vi "HW XML Tx - Write.vi"(0 "String (in)":string, 7 "Parameter Array":T1[](array[typedef])) -> (4 "String (out)":string)   [LabVIEW 2017]
uses:
  Controls/Database_Array.ctl
  Controls/Encoding.ctl
  <userlib>/_OpenG.lib/array/array.llb/Remove Duplicates from 1D Array (I32)__ogtk.vi
  <userlib>/_OpenG.lib/array/array.llb/Filter 1D Array with Scalar (I32)__ogtk.vi
  <userlib>/_OpenG.lib/array/array.llb/Index 1D Array Elements (Variant)__ogtk.vi
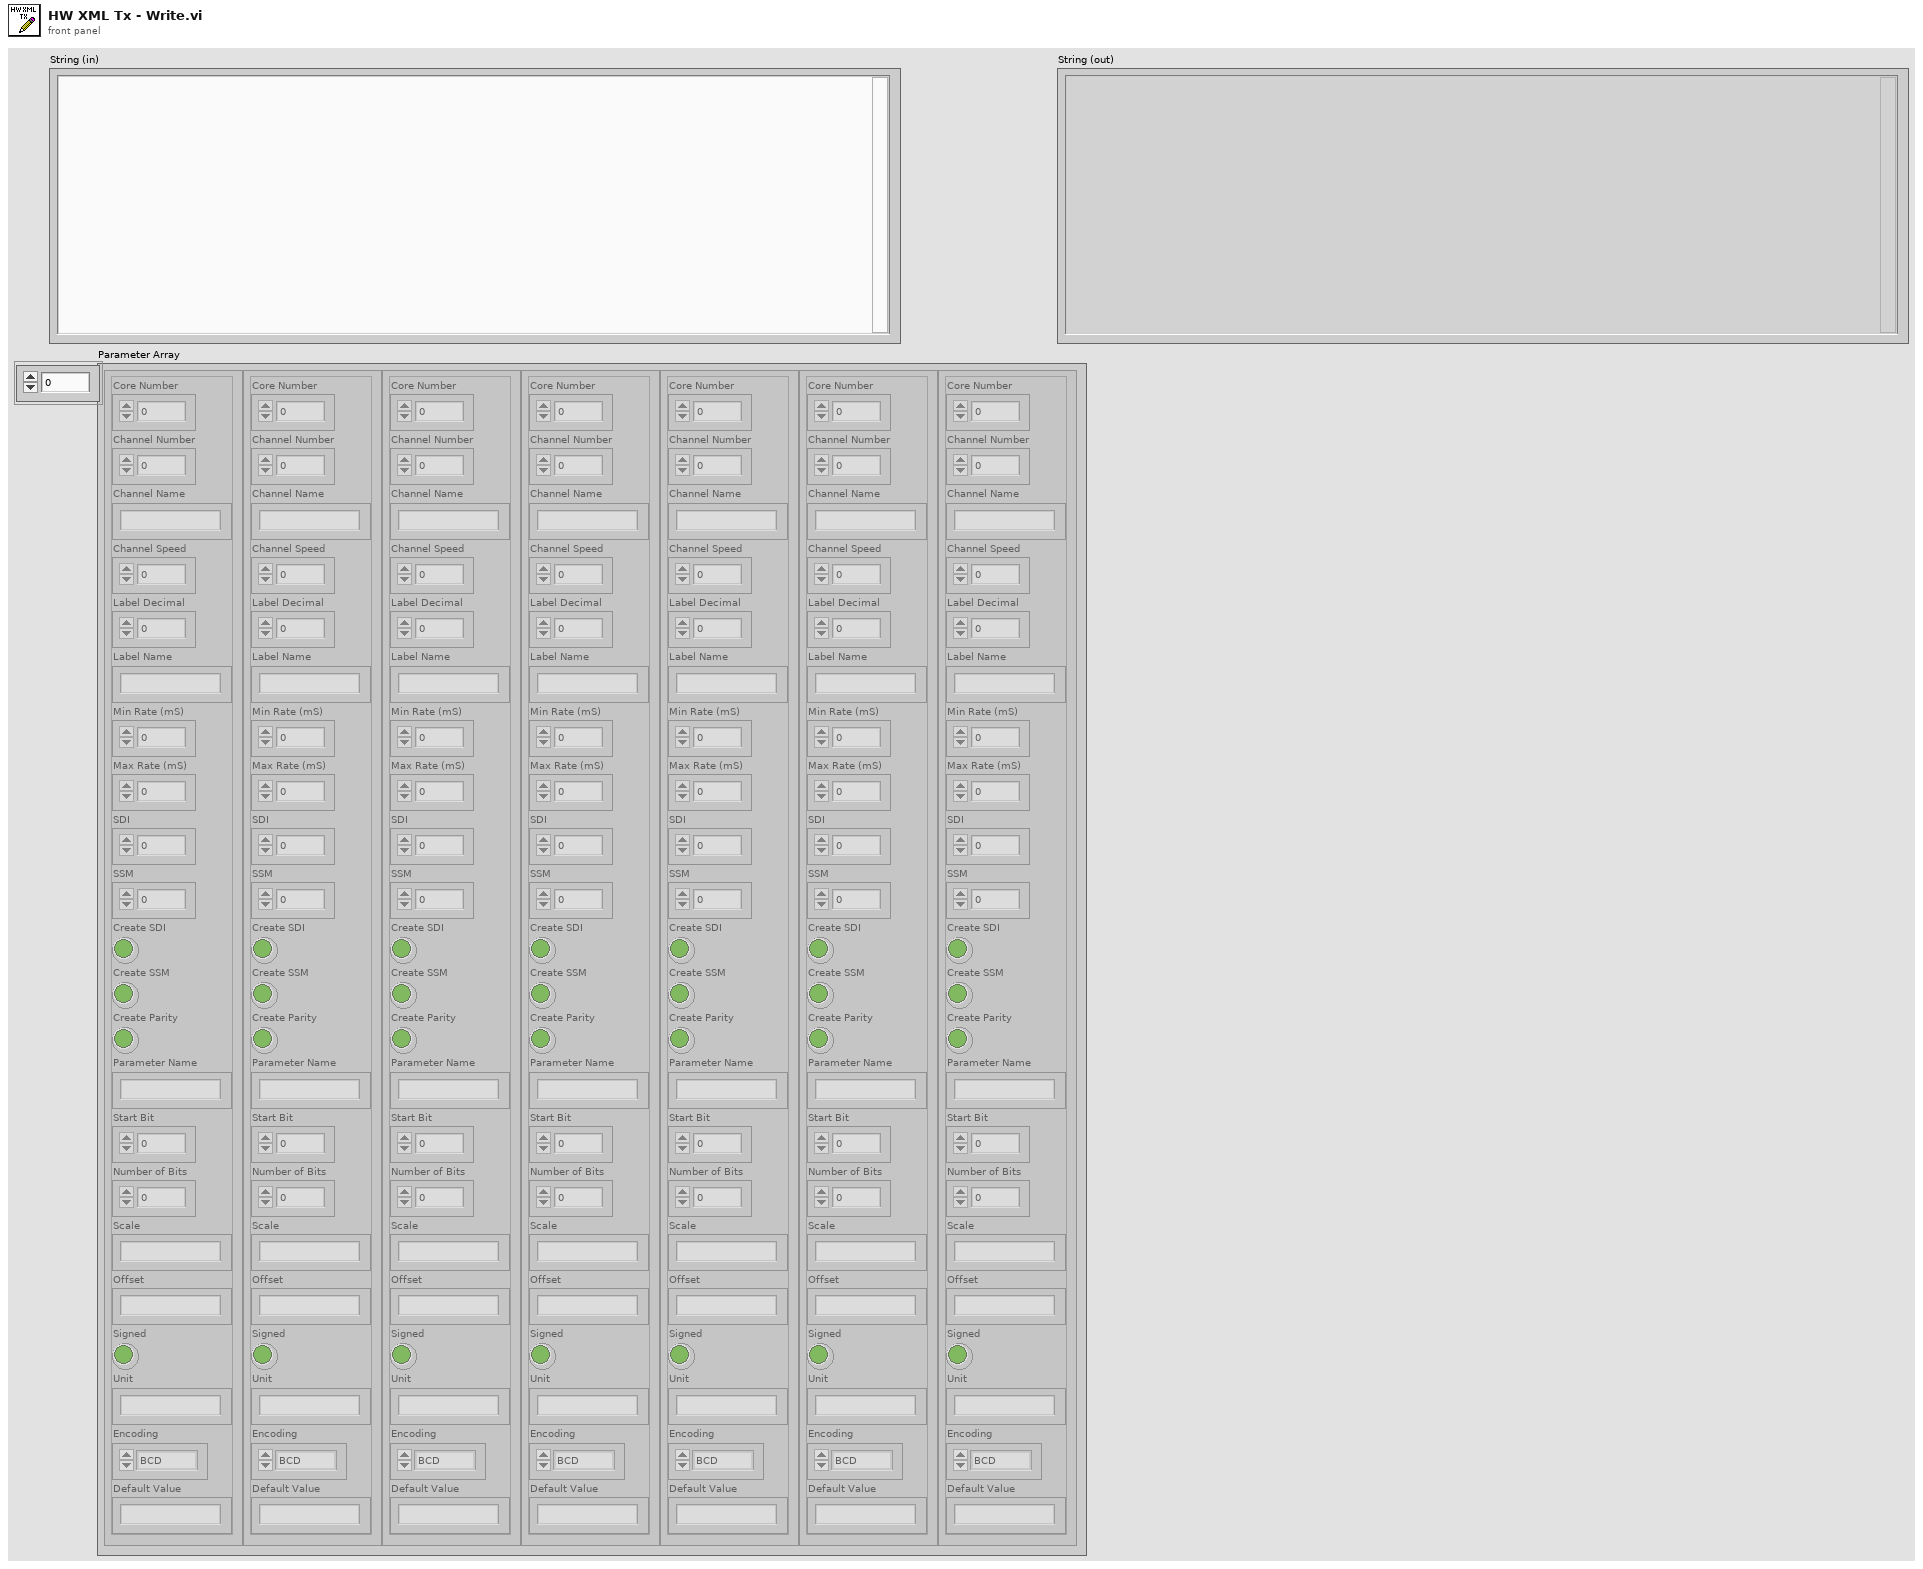
[diagram p1: front panel]
types:
  T1 = typedef "Database_Array.ctl" = cluster{"Core Number":i32, "Channel Number":i32, "Channel Name":string, "Channel Speed":i32, "Label Decimal":i32, "Label Name":string, "Min Rate (mS)":i32, "Max Rate (mS)":i32, "SDI":i32, "SSM":i32, "Create SDI":bool, "Create SSM":bool, "Create Parity":bool, "Parameter Name":string, "Start Bit":i32, "Number of Bits":i32, "Scale":string, "Offset":string, "Signed":bool, "Unit":string, "Encoding":T2, "Default Value":string}
  T2 = typedef "Encoding.ctl" = enum16{"BCD", "BNR", "Discrete"}
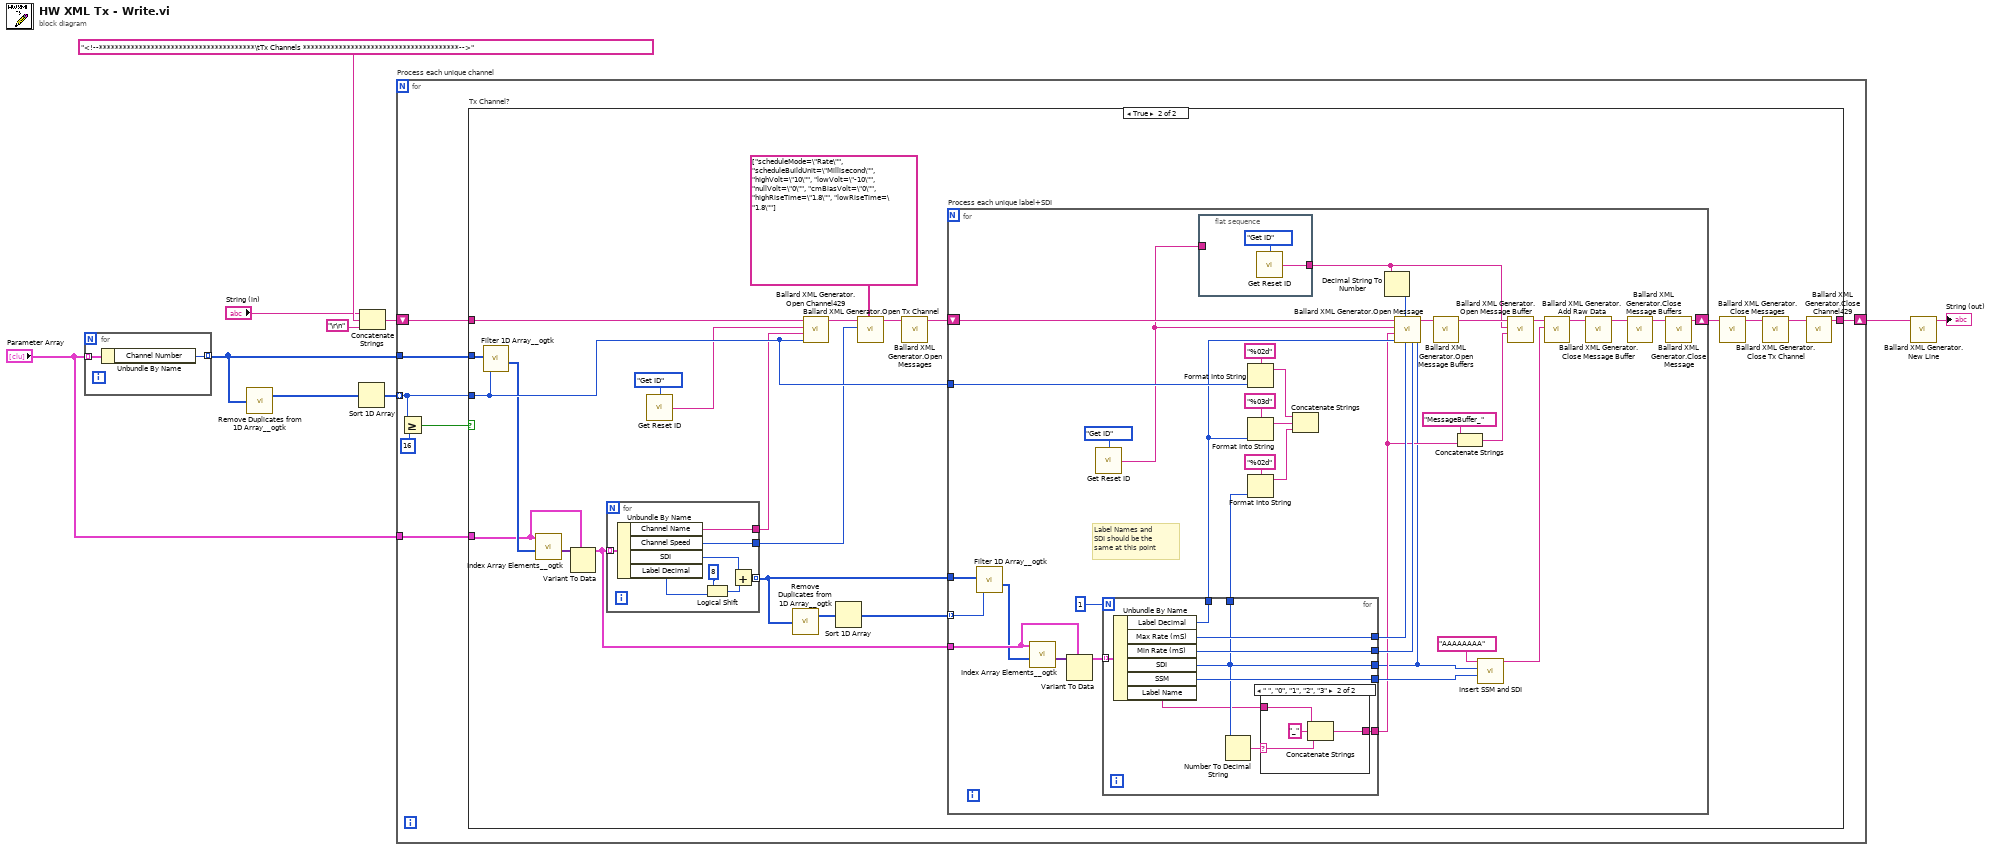
[diagram p0: block diagram]
diagram:
  n1 = for {
    tunnel: [w12] -> w2 mode=indexing
    tunnel: "Parameter Array" -> [w11] mode=indexing
    n2 = Unbundle By Name(w11) -> ("Channel Number"=w12:i32)
  }
  n3 = call-poly <userlib>:"Remove Duplicates from 1D Array__ogtk.vi"("Input Array"=w2) -> ("Output Array"=w9:i32[])  [unwired: 1 out]
  n4 = Sort 1D Array(array=w9) -> (sorted array=w10:i32[])
  n5 = Concatenate Strings("String (in)", "<!--***************************************\tTx Channels ***************************************-->", "\r\n") -> (w6:string)
  n6 = for "Process each unique channel" {
    tunnel: w10 -> [w16] mode=indexing
    tunnel: w2 -> [w19]
    shift-right: [w17] -> w1
    shift-left: w6 -> [w18]
    tunnel: "Parameter Array" -> [w13]
    n7 = Greater Or Equal?(x=w16, y=16) -> (x >= y?=w15:bool)
    n8 = case "Tx Channel?" shown="True" w15 {
      tunnel: w19 -> [_ w42]
      tunnel: w18 -> [w20 w39]
      tunnel: [w20 w32] -> w17
      tunnel: w16 -> [_ w31]
      tunnel: w13 -> [_ w25]
      frame False {
      }
      frame True {
        n9 = call-poly <userlib>:"Filter 1D Array__ogtk.vi"("items to filter"=w31, "array"=w42) -> ("filtered item indices"=w29:i32[])  [unwired: 4 in, 1 out]
        n10 = call-poly <userlib>:"Index Array Elements__ogtk.vi"("indices"=w29, "array"=w25) -> ("elements"=w28:variant[])  [unwired: 9 in]
        n11 = Variant To Data(type=w25, Variant=w28) -> (data=w24:T1[])  [unwired: 1 in, 1 out]
        n12 = for {
          tunnel: w24 -> [w50] mode=indexing
          tunnel: [w49] -> w27
          tunnel: [w48] -> w26
          tunnel: [w43] -> w23 mode=indexing
          n13 = Unbundle By Name(w50) -> ("Channel Name"=w49:string, "Channel Speed"=w48:i32, "SDI"=w45:i32, "Label Decimal"=w44:i32)
          n14 = Logical Shift(y=i16 8, x=w44) -> (x << y=w47:i32)
          n15 = Add(x=w45, y=w47) -> (x+y=w43:i32)
        }
        n16 = call "Get Reset ID.vi"("Function"=enum16{"Get ID", "Reset ID"}."Get ID") -> ("ID"=w22:string)  [unwired: 14 in]
        n17 = call-poly <userlib>:"Remove Duplicates from 1D Array__ogtk.vi"("Input Array"=w23) -> ("Output Array"=w41:i32[])  [unwired: 1 out]
        n18 = call "Ballard XML Generator.Open Channel429.vi"("hardware channel"=w31, "name"=w27, "id"=w22, "string in"=w39) -> ("string out"=w37:string)  [unwired: 7 in]
        n19 = Sort 1D Array(array=w41) -> (sorted array=w40:i32[])
        n20 = call "Ballard XML Generator.Open Tx Channel.vi"("other params"=string[] ["scheduleMode=\"Rate\"", "scheduleBuildUnit=\"Millisecond\"", "highVolt=\"10\"", "lowVolt=\"-10\"", "nullVolt=\"0\"", "cmBiasVolt=\"0\"", "highRiseTime=\"1.8\"", "lowRiseTime=\"1.8\""], "speedKHz"=w26, "string in"=w37) -> ("string out"=w38:string)  [unwired: 8 in]
        n21 = call "Ballard XML Generator.Open Messages.vi"("string in"=w38) -> ("string out"=w36:string)  [unwired: 10 in]
        n22 = for "Process each unique label+SDI" {
          tunnel: w40 -> [w83] mode=indexing
          tunnel: w23 -> [w87]
          shift-right: [w71] -> w35
          shift-left: w36 -> [w86]
          tunnel: w24 -> [w64]
          tunnel: w31 -> [w82]
          # "Label Names and SDI should be the same at this point"
          n23 = call-poly <userlib>:"Filter 1D Array__ogtk.vi"("items to filter"=w83, "array"=w87) -> ("filtered item indices"=w63:i32[])  [unwired: 4 in, 1 out]
          n24 = call-poly <userlib>:"Index Array Elements__ogtk.vi"("indices"=w63, "array"=w64) -> ("elements"=w67:variant[])  [unwired: 9 in]
          n25 = Variant To Data(type=w64, Variant=w67) -> (data=w66:T1[])  [unwired: 1 in, 1 out]
          n26 = call "Get Reset ID.vi"("Function"=enum16{"Get ID", "Reset ID"}."Get ID") -> ("ID"=w51:string)  [unwired: 14 in]
          n27 = for {
            N: 1 -> [_]
            tunnel: w66 -> [w98] mode=indexing
            tunnel: [w97] -> w62
            tunnel: [w96] -> w61
            tunnel: [w92] -> w54
            tunnel: [w95] -> w60
            tunnel: [w94] -> w59
            tunnel: [w92] -> w56
            tunnel: [w93] -> w55
            n28 = Unbundle By Name(w98) -> ("Label Decimal"=w94:i32, "Max Rate (mS)"=w97:i32, "Min Rate (mS)"=w96:i32, "SDI"=w92:i32, "SSM"=w95:i32, "Label Name"=w91:string)
            n29 = Number To Decimal String(number=w92) -> (decimal integer string=w90:string)  [unwired: 1 in]
            n30 = case shown="\" \", \"0\", \"1\", \"2\", \"3\"" w90 {
              selector: w90 -> [_ w100]
              tunnel: [w99 w103] -> w93
              tunnel: w91 -> [w99 w101]
              frame "Default", Default {
              }
              frame " ", "0", "1", "2", "3" {
                n31 = Concatenate Strings(w101, "_" ("string"), w100) -> (w103:string)
              }
            }
          }
          n32 = flat-sequence {
            tunnel: [w89] -> w52
            tunnel: w51 -> [_]
            frame #0 {
              n33 = call "Get Reset ID.vi"("Function"=enum16{"Get ID", "Reset ID"}."Get ID") -> ("ID"=w89:string)  [unwired: 14 in]
            }
          }
          n34 = Format Into String(format string="%02d", w82) -> (resulting string=w81:string)  [unwired: 2 in, 1 out]
          n35 = Format Into String(format string="%03d", w59) -> (resulting string=w80:string)  [unwired: 2 in, 1 out]
          n36 = Format Into String(format string="%02d", w56) -> (resulting string=w57:string)  [unwired: 2 in, 1 out]
          n37 = Concatenate Strings(w81, w80, w57) -> ()  [unwired: 1 out]
          n38 = Decimal String To Number(string=w52) -> (number=w70:i32)  [unwired: 2 in, 1 out]
          n39 = call "Ballard XML Generator.Open Message.vi"("SDI"=w54, "minRate (400)"=w61, "maxRate (400)"=w62, "messageBufferIDRef (128)"=w70, "labelDecimal"=w59, "name"=w55, "id"=w51, "string in"=w86) -> ("string out"=w79:string)  [unwired: 3 in]
          n40 = call "Ballard XML Generator.Open Message Buffers.vi"("string in"=w79) -> ("string out"=w78:string)  [unwired: 10 in]
          n41 = Concatenate Strings("MessageBuffer_" ("name"), w55) -> (w76:string)
          n42 = call "Insert SSM and SDI.vi"("SSM"=w60, "SDI"=w54, "Hex (in)"="AAAAAAAA" ("raw data")) -> ("Hex (out)"=w68:string)  [unwired: 8 in]
          n43 = call "Ballard XML Generator.Open Message Buffer.vi"("name"=w76, "id"=w52, "string in"=w78) -> ("string out"=w72:string)  [unwired: 8 in]
          n44 = call "Ballard XML Generator.Add Raw Data.vi"("raw data"=w68, "string in"=w72) -> ("string out"=w73:string)  [unwired: 9 in]
          n45 = call "Ballard XML Generator.Close Message Buffer.vi"("string in"=w73) -> ("string out"=w74:string)  [unwired: 10 in]
          n46 = call "Ballard XML Generator.Close Message Buffers.vi"("string in"=w74) -> ("string out"=w75:string)  [unwired: 10 in]
          n47 = call "Ballard XML Generator.Close Message.vi"("string in"=w75) -> ("string out"=w71:string)  [unwired: 10 in]
        }
        n48 = call "Ballard XML Generator.Close Messages.vi"("string in"=w35) -> ("string out"=w34:string)  [unwired: 10 in]
        n49 = call "Ballard XML Generator.Close Tx Channel.vi"("string in"=w34) -> ("string out"=w33:string)  [unwired: 10 in]
        n50 = call "Ballard XML Generator.Close Channel429.vi"("string in"=w33) -> ("string out"=w32:string)  [unwired: 10 in]
      }
    }
  }
  n51 = call "Ballard XML Generator.New Line.vi"("string in"=w1) -> ("string out"=→"String (out)":string)  [unwired: 10 in]
